vi "To B&W, Remove Particle (Main SubVI).vi"(7 "Image Reference Sources":T2, 8 "error in (no error)":errorcluster, 10 "Number of Erosion":i32=2, 11 "Refnum in":T1) -> (0 "error out":errorcluster, 1 "Number of Particles after":i32, 2 "Image Out":T1, 3 "Current Grayscale":T1, 4 "Original":T1(plugin-control), 5 "Number of Particles before":i32, 6 "Cluster":T3)   [LabVIEW 2014]
uses:
  <vilib>/vision/Image Controls.llb/IMAQ Image.ctl
  <vilib>/vision/NI_Vision_Development_Module.lvlib
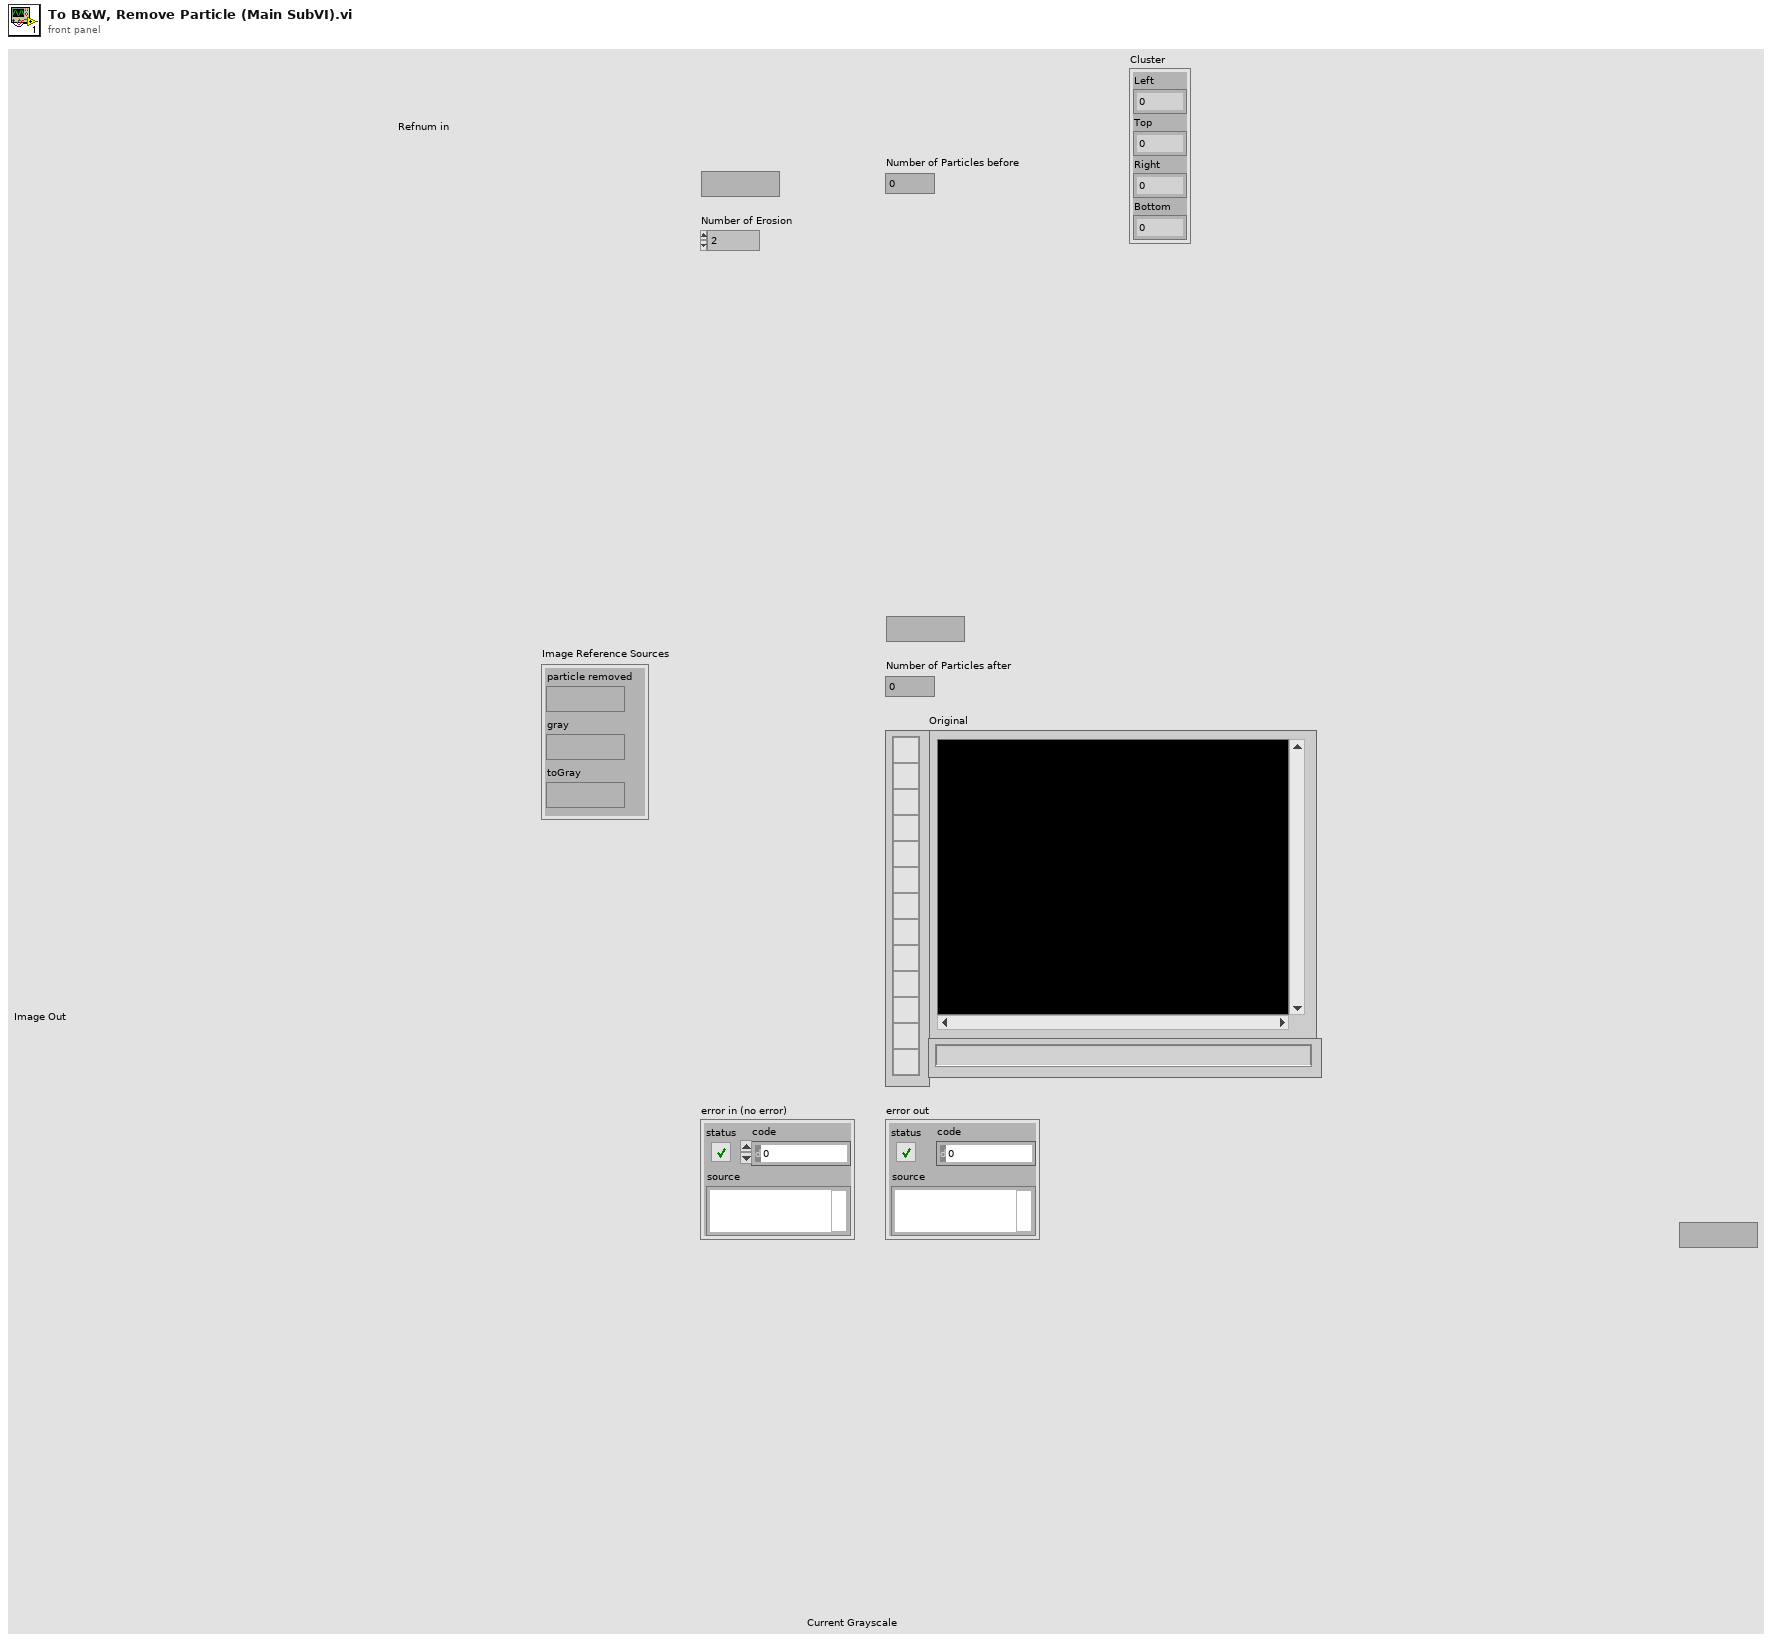
[diagram p1: front panel]
types:
  T1 = typedef "IMAQ Image.ctl" = refnum<image>
  T2 = cluster{"particle removed":T1, "gray":T1, "toGray":T1}
  T3 = cluster{"Left":dbl, "Top":dbl, "Right":dbl, "Bottom":dbl}
  T4 = typedef "Particle Parameters" = i32
  T5 = typedef "Image Type" = u32
  T6 = cluster{"Numeric":dbl, "Numeric":dbl, "Numeric":dbl, "Numeric":dbl}
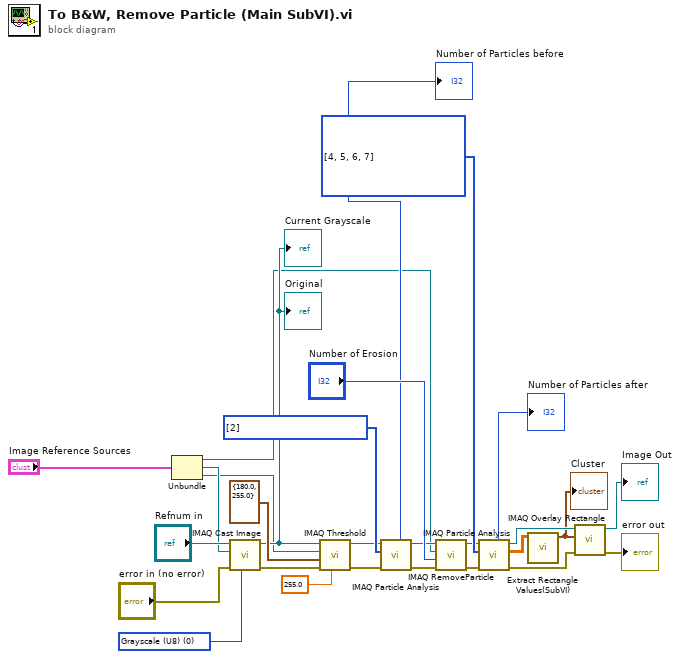
[diagram p0: block diagram]
diagram:
  w23 = T4[] [4, 5, 6, 7] items=["Center of Mass X", "Center of Mass Y", "First Pixel X", "First Pixel Y", "Bounding Rect Left", "Bounding Rect Top", "Bounding Rect Right", "Bounding Rect Bottom", "Max Feret Diameter Start X", "Max Feret Diameter Start Y", "Max Feret Diameter End X", "Max Feret Diameter End Y", "Max Horiz. Segment Length Left", "Max Horiz. Segment Length Right", "Max Horiz. Segment Length Row", "-", "Bounding Rect Width", "Bounding Rect Height", "Bounding Rect Diagonal", "Perimeter", "Convex Hull Perimeter", "Holes' Perimeter", "Max Feret Diameter", "Equivalent Ellipse Major Axis", "Equivalent Ellipse Minor Axis", "Equivalent Ellipse Minor Axis (Feret)", "Equivalent Rect Long Side", "Equivalent Rect Short Side", "Equivalent Rect Diagonal", "Equivalent Rect Short Side (Feret)", "Average Horiz. Segment Length", "Average Vert. Segment Length", "Hydraulic Radius", "Waddel Disk Diameter", "-", "Area", "Holes' Area", "Particle & Holes' Area", "Convex Hull Area", "Image Area", "-", "Number of Holes", "Number of Horiz. Segments", "Number of Vert. Segments", "-", "Orientation", "Max Feret Diameter Orientation", "-", "% Area/Image Area", "% Area/(Particle & Holes' Area)", "Ratio of Equivalent Ellipse Axes", "Ratio of Equivalent Rect Sides", "-", "Elongation Factor", "Compactness Factor", "Heywood Circularity Factor", "Type Factor", "-", "Sum X", "Sum Y", "Sum XX", "Sum XY", "Sum YY", "Sum XXX", "Sum XXY", "Sum XYY", "Sum YYY", "-", "Moment of Inertia XX", "Moment of Inertia XY", "Moment of Inertia YY", "Moment of Inertia XXX", "Moment of Inertia XXY", "Moment of Inertia XYY", "Moment of Inertia YYY", "Norm. Moment of Inertia XX", "Norm. Moment of Inertia XY", "Norm. Moment of Inertia YY", "Norm. Moment of Inertia XXX", "Norm. Moment of Inertia XXY", "Norm. Moment of Inertia XYY", "Norm. Moment of Inertia YYY", "Hu Moment 1", "Hu Moment 2", "Hu Moment 3", "Hu Moment 4", "Hu Moment 5", "Hu Moment 6", "Hu Moment 7"] ("Pixel Measurements")
  w13 = T4[] [2] items=["Center of Mass X", "Center of Mass Y", "First Pixel X", "First Pixel Y", "Bounding Rect Left", "Bounding Rect Top", "Bounding Rect Right", "Bounding Rect Bottom", "Max Feret Diameter Start X", "Max Feret Diameter Start Y", "Max Feret Diameter End X", "Max Feret Diameter End Y", "Max Horiz. Segment Length Left", "Max Horiz. Segment Length Right", "Max Horiz. Segment Length Row", "-", "Bounding Rect Width", "Bounding Rect Height", "Bounding Rect Diagonal", "Perimeter", "Convex Hull Perimeter", "Holes' Perimeter", "Max Feret Diameter", "Equivalent Ellipse Major Axis", "Equivalent Ellipse Minor Axis", "Equivalent Ellipse Minor Axis (Feret)", "Equivalent Rect Long Side", "Equivalent Rect Short Side", "Equivalent Rect Diagonal", "Equivalent Rect Short Side (Feret)", "Average Horiz. Segment Length", "Average Vert. Segment Length", "Hydraulic Radius", "Waddel Disk Diameter", "-", "Area", "Holes' Area", "Particle & Holes' Area", "Convex Hull Area", "Image Area", "-", "Number of Holes", "Number of Horiz. Segments", "Number of Vert. Segments", "-", "Orientation", "Max Feret Diameter Orientation", "-", "% Area/Image Area", "% Area/(Particle & Holes' Area)", "Ratio of Equivalent Ellipse Axes", "Ratio of Equivalent Rect Sides", "-", "Elongation Factor", "Compactness Factor", "Heywood Circularity Factor", "Type Factor", "-", "Sum X", "Sum Y", "Sum XX", "Sum XY", "Sum YY", "Sum XXX", "Sum XXY", "Sum XYY", "Sum YYY", "-", "Moment of Inertia XX", "Moment of Inertia XY", "Moment of Inertia YY", "Moment of Inertia XXX", "Moment of Inertia XXY", "Moment of Inertia XYY", "Moment of Inertia YYY", "Norm. Moment of Inertia XX", "Norm. Moment of Inertia XY", "Norm. Moment of Inertia YY", "Norm. Moment of Inertia XXX", "Norm. Moment of Inertia XXY", "Norm. Moment of Inertia XYY", "Norm. Moment of Inertia YYY", "Hu Moment 1", "Hu Moment 2", "Hu Moment 3", "Hu Moment 4", "Hu Moment 5", "Hu Moment 6", "Hu Moment 7"] ("Pixel Measurements")
  w9 = T5 0 items=["Grayscale (U8)", "Grayscale (I16)", "Grayscale (SGL)", "Complex (CSG)", "RGB (U32)", "HSL (U32)", "RGB (U64)", "Grayscale (U16)"] ("Image Type")
  n1 = Unbundle("Image Reference Sources") -> ("particle removed"=w4:T1, "gray"=w3:T1, "toGray"=w2:T1)
  n2 = call "IMAQ Cast Image"("Image Type"=w9, "error in (no error)"="error in (no error)", "Image Dst"=w3, "Image Src"="Refnum in") -> ("error out"=w12:errorcluster, "Image Dst Out"=w6:T1)  [unwired: 6 in]
  "Original" <- w6
  "Current Grayscale" <- w6
  n3 = call "IMAQ Threshold"("Replace Value"=sgl 255.0, "error in (no error)"=w12, "Range"=cluster{"Lower value":sgl, "Upper value":sgl} {"Lower value"=180.0, "Upper value"=255.0}, "Image Dst"=w2, "Image Src"=w6) -> ("error out"=w15:errorcluster, "Image Dst Out"=w7:T1)  [unwired: 5 in]
  n4 = call "IMAQ Particle Analysis"("error in (no error)"=w15, "Pixel Measurements"=w13, "Image"=w7) -> ("error out"=w18:errorcluster, "Image Out (duplicate)"=w16:T1, "Number of Particles"=→"Number of Particles before":i32)  [unwired: 3 in, 3 out]
  n5 = call "IMAQ RemoveParticle"("error in (no error)"=w18, "Number of Erosion"="Number of Erosion", "Image Dst"=w4, "Image Src"=w16) -> ("error out"=w21:errorcluster, "Image Dst Out"=w22:T1)  [unwired: 6 in]
  n6 = call "IMAQ Particle Analysis"("error in (no error)"=w21, "Pixel Measurements"=w23, "Image"=w22) -> ("error out"=w28:errorcluster, "Particle Measurements (Pixels)"=w24:dbl[][], "Image Out (duplicate)"=w26:T1, "Number of Particles"=→"Number of Particles after":i32)  [unwired: 3 in, 2 out]
  n7 = call "Extract Rectangle Values(SubVI).vi"("Particle Measurements (Pixels)"=w24) -> ("Cluster"=w1:T6)  [unwired: 10 in]
  "Cluster" <- w1
  n8 = call "IMAQ Overlay Rectangle"("error in (no error)"=w28, "Rectangle"=w1, "Image"=w26) -> ("error out"=→"error out":errorcluster, "Image Out"=→"Image Out":T1)  [unwired: 7 in]
